vi "写入excel.vi"(6 "Item":string, 7 "Measurement":dbl, 8 "error in (no error)":errorcluster, 10 "Arguments":string[](array[string]), 11 "NI_report输入":refnum<class "NI_report.lvclass">) -> (0 "error out":errorcluster, 3 "report out":refnum<class "NI_report.lvclass">)   [LabVIEW 2020]
uses:
  <vilib>/Utility/NIReport.llb/NI_report.lvclass
  <vilib>/addons/_office/_exclsub.llb/font.ctl
  <vilib>/Utility/NIReport.llb/Excel/NI_Excel.lvclass
  <vilib>/addons/_office/NI_ReportGenerationToolkit.lvlib
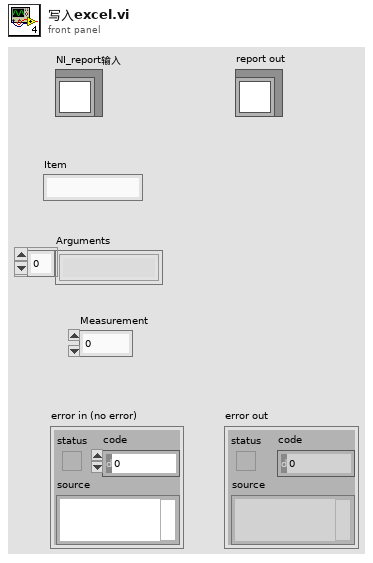
[diagram p1: front panel]
types:
  T1 = typedef "NI_ReportGenerationToolkit.lvlib/font.ctl" = cluster{"font name":string, "font size":dbl, "bold":u16, "italic":u16, "underline":u16, "strike through":u16, "font color":u32}
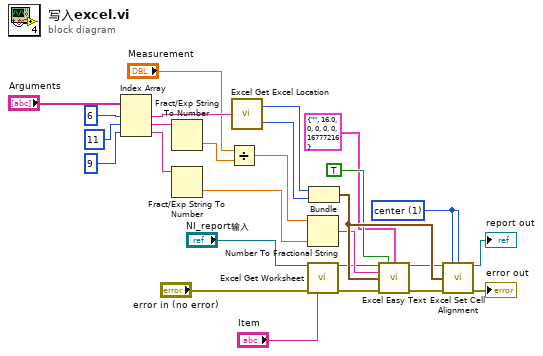
[diagram p0: block diagram]
diagram:
  w26 = 1 items=["top", "center", "bottom"] ("vertical alignment (top)")
  n1 = Index Array(array="Arguments", index #1=6 ("索引 (行)"), index #2=11 ("索引 (行)"), index #3=9 ("索引 (行)")) -> (element #1=w19:string, element #2=w14:string, element #3=w20:string)
  n2 = Fract/Exp String To Number(string=w14) -> (number=w15:dbl)  [unwired: 3 in, 1 out]
  n3 = Fract/Exp String To Number(string=w20) -> (number=w21:dbl)  [unwired: 3 in, 1 out]
  n4 = Divide(x="Measurement", y=w15) -> (x/y=w17:dbl)
  n5 = call <vilib>:"Excel Get Excel Location.vi"("cell's name"=w19) -> ("row"=w22:i32, "column"=w23:i32)
  n6 = Number To Fractional String(number=w17, precision (6)=w21) -> (F-format string=w18:string)  [unwired: 2 in]
  n7 = call <vilib>:"Excel Get Worksheet.vi"("report in"="NI_report输入", "error in (no error)"="error in (no error)", "name (\"\")"="Item") -> ("report out"=w7:refnum<class "NI_report.lvclass">, "error out"=w6:errorcluster)  [unwired: 11 in]
  n8 = Bundle("row"=w22, "column"=w23) -> (w27:cluster{"row":i32, "column":i32})  [unwired: 1 in]
  n9 = call <vilib>:"Excel Easy Text.vi"("report in"=w7, "border? (F)"=TRUE, "font"=T1 {"font name"="", "font size"=16.0, "bold"=0, "italic"=0, "underline"=0, "strike through"=0, "font color"=16777216}, "text"=w18, "start (-1, -1)"=w27, "error in (no error)"=w6) -> ("report out"=w25:refnum<class "NI_report.lvclass">, "error out"=w24:errorcluster)  [unwired: 5 in, 3 out]
  n10 = call <vilib>:"Excel Set Cell Alignment.vi"("report in"=w25, "vertical alignment (top)"=w26, "horizontal alignment (left)"=w26, "start (-1, -1)"=w27, "error in (no error)"=w24) -> ("report out"=→"report out":refnum<class "NI_report.lvclass">, "error out"=→"error out":errorcluster)  [unwired: 9 in]
